vi "Analyse Content.vi"(8 "error in (no error)":errorcluster, 11 "Text in":refnum<class "Text.lvclass">) -> (0 "error out":errorcluster, 3 "Text out":refnum<class "Text.lvclass">)   [LabVIEW 2026, in "LED Matrix.lvlib" / "Text.lvclass"]
uses:
  Text.lvclass
  home/pete/dev/labview-car/dev/LED Matrix/Content/Content.lvclass
  Text.lvclass/Text.ctl
  Content/Content.lvclass
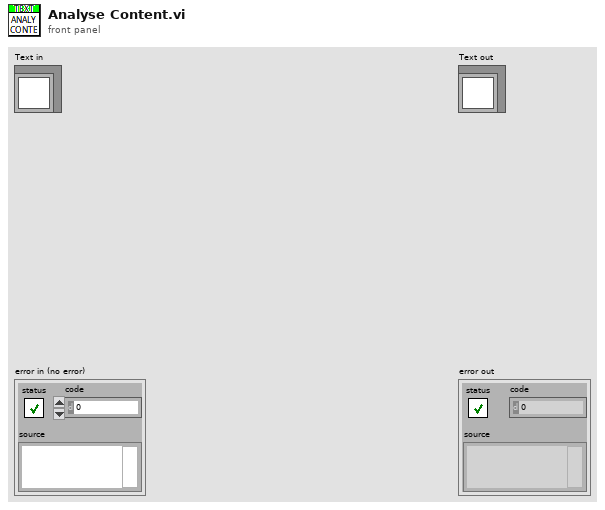
[diagram p1: front panel]
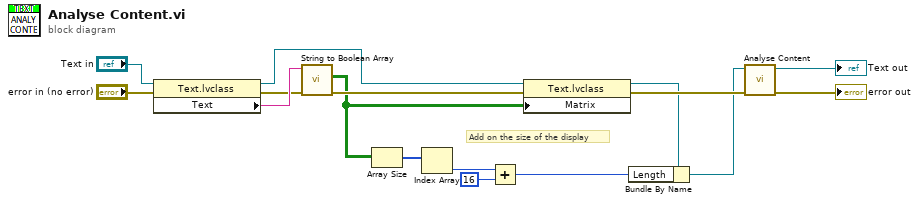
[diagram p0: block diagram]
diagram:
  # "Add on the size of the display"
  n1 = property class="Text.lvclass"(reference="Text in", error in="error in (no error)") -> (reference out=w10:refnum<class "Text.lvclass">, error out=w12:errorcluster, "Text"=w14:string)
  n2 = call "String to Boolean Array.vi"("error in (no error)"=w12, "String"=w14) -> ("error out"=w13:errorcluster, "Array"=w6:bool[][])  [unwired: 8 in]
  n3 = Array Size(array=w6) -> (size(s)=w5:i32[])
  n4 = Index Array(array=w5) -> (element=w3:i32)  [unwired: 1 in]
  n5 = Add(x=w3, y=16) -> (x+y=w1:i32)
  n6 = property class="Text.lvclass"(reference=w10, error in=w13, "Matrix"=w6) -> (reference out=w8:refnum<class "Text.lvclass">, error out=w11:errorcluster)
  n7 = Bundle By Name(cluster=w8, "Length"=w1) -> (w4:refnum<class "Text.lvclass">)
  n8 = call-parent "Analyse Content.vi"("error in (no error)"=w11, "Content in"=w4) -> ("error out"=→"error out":errorcluster, "Content out"=→"Text out":refnum<class "Text.lvclass">)  [unwired: 8 in]
